vi "subscribe single data.vi"(8 "error in":errorcluster, 10 "subscription command":string, 11 "refnum in":T1) -> (0 "error out":errorcluster, 3 "refnum in":T1)   [LabVIEW 2023, in "Publisher Subscriber.lvlib"]
uses:
  <userlib>/_Publisher Subscriber/Publisher Subscriber.lvlib
  <userlib>/_Publisher Subscriber/Controls/node refnum.ctl
  <userlib>/_Publisher Subscriber/Controls/node dvr data.ctl
  <userlib>/_Publisher Subscriber/Controls/data cluster.ctl
  <userlib>/_Publisher Subscriber/Controls/subscription bank ref.ctl
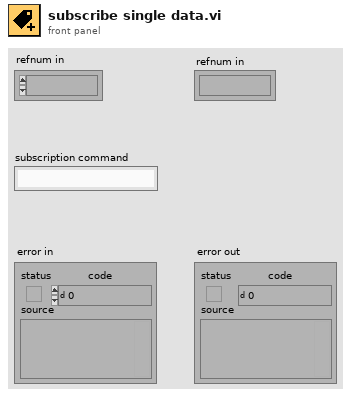
[diagram p1: front panel]
types:
  T1 = typedef "Publisher Subscriber.lvlib/node refnum.ctl" = refnum<vi>
  T2 = typedef "Publisher Subscriber.lvlib/node dvr data.ctl" = cluster{"queue ref":refnum<queue>, "Subscription Bank Ref":refnum<data-value>, "Command":string, "Data":variant, "Subscriptions []":set{string}, "Variables DVR Ref":refnum<data-value>}
  T3 = typedef "Publisher Subscriber.lvlib/subscription bank ref.ctl" = map{string, set{refnum<queue>}}
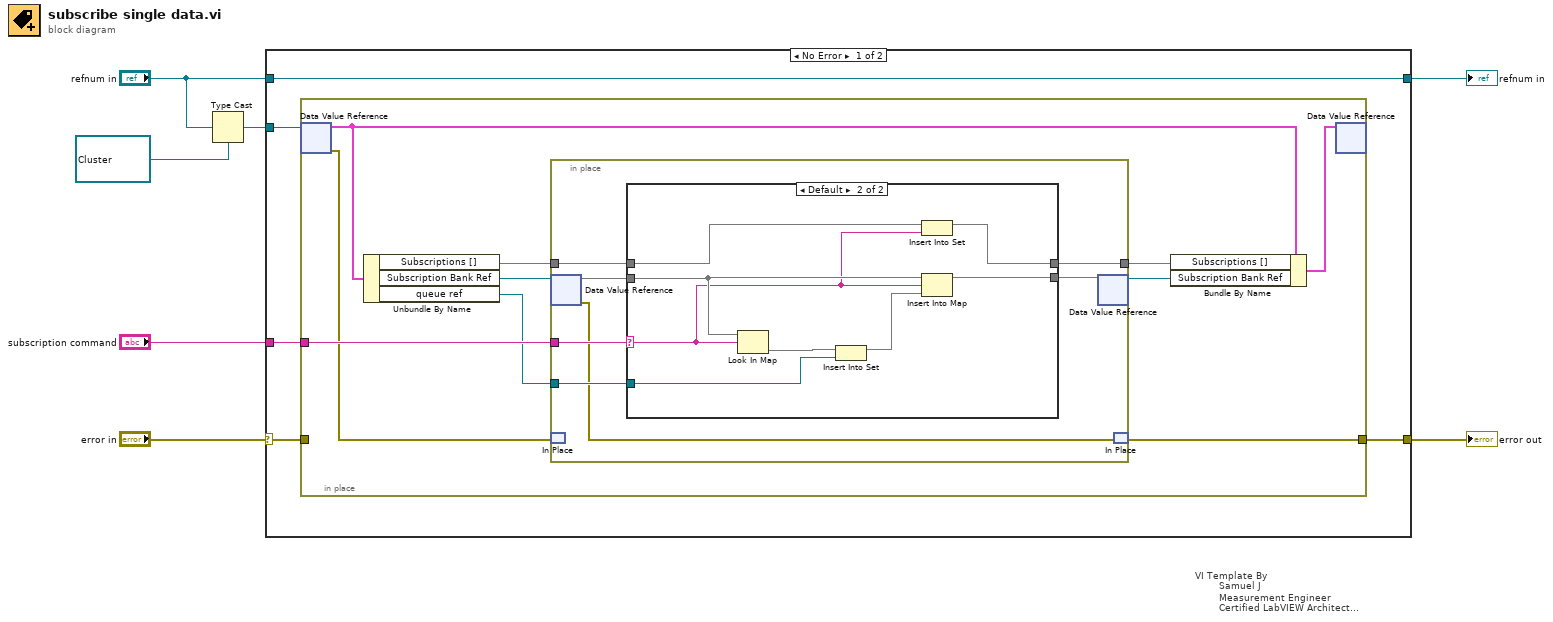
[diagram p0: block diagram]
diagram:
  n1 = Type Cast(type=refnum<data-value> refnum ("data value reference"), x="refnum in") -> (*(type *) &x=w3:refnum<data-value>)
  n2 = case "VI Template By\n        Samuel J\n        Measurement Engineer\n        Certified LabVIEW Architect\n        Vestas Technology R&D Chennai" shown="No Error" "error in" {
    selector: "error in" -> [w9 w41]
    tunnel: [w8 w41] -> w6
    tunnel: "subscription command" -> [w10 _]
    tunnel: w3 -> [w11 _]
    tunnel: [w12 w40] -> w2
    tunnel: "refnum in" -> [w12 w40]
    frame No Error {
      n3 = in-place {
        in-place-border: w10 -> [w19]
        in-place-border: [w14] -> w8
        in-place-border: w9 -> [_]
        n4 = in-place-dvr #1(w11) -> (w21:T2, w13:errorcluster)
        n5 = Unbundle By Name(w21) -> ("Subscriptions []"=w16:set{string}, "Subscription Bank Ref"=w20:refnum<data-value>, "queue ref"=w17:refnum<queue>)
        n6 = in-place {
          in-place-border: w19 -> [w26]
          in-place-border: w17 -> [w27]
          in-place-border: w16 -> [w25]
          in-place-border: [w24] -> w15
          n7 = in-place-dvr #2(w20) -> (w29:T3, w23:errorcluster)
          n8 = in-place-match #3(w13) -> ()  [unwired: 1 out]
          n9 = case shown="Default" w26 {
            selector: w26 -> [_ w35]
            tunnel: w29 -> [w30 w38]
            tunnel: [w30 w37] -> w28
            tunnel: w27 -> [_ w36]
            tunnel: w25 -> [w31 w34]
            tunnel: [w31 w33] -> w24
            frame "" {
            }
            frame Default {
              n10 = Look In Map(map=w38, key=w35) -> (value=w39:set{refnum<queue>})  [unwired: 1 in, 1 out]
              n11 = Insert Into Set(10:w36, 11:w39) -> (3:w32:set{refnum<queue>})  [unwired: 1 out]
              n12 = Insert Into Set(10:w35, 11:w34) -> (3:w33:set{string})  [unwired: 1 out]
              n13 = Insert Into Map(map in=w38, key=w35, value=w32) -> (map out=w37:T3)  [unwired: 2 out]
            }
          }
          n14 = in-place-dvr #2(w28) -> (w18:refnum<data-value>)  [unwired: 1 out]
          n15 = in-place-match #3(w23) -> (w14:errorcluster)
        }
        n16 = Bundle By Name(cluster=w21, "Subscriptions []"=w15, "Subscription Bank Ref"=w18) -> (w22:T2)
        n17 = in-place-dvr #1(w22) -> ()  [unwired: 2 out]
      }
    }
    frame Error {
    }
  }
  "error out" <- w6
  "refnum in" <- w2
